vi "EnableCell.vi"(0 "SingleValMenuCol in":refnum<class "SingleValMenuCol.lvclass">, 5 "Cell Position":T1, 7 "Table Data in":string[][](array[string]), 9 "Table CtlRef In":refnum<vi>, 11 "error in (no error)":errorcluster) -> (4 "SingleValMenuCol out":refnum<class "SingleValMenuCol.lvclass">, 8 "Table Data out":string[][](array[string]), 10 "Table CtlRef Out":refnum<vi>, 15 "error out":errorcluster)   [LabVIEW 2013, in "SingleValMenuCol.lvclass"]
uses:
  SingleValMenuCol.lvclass
  <vilib>/Utility/miscctls.llb/LVRowAndColumnTypeDef.ctl
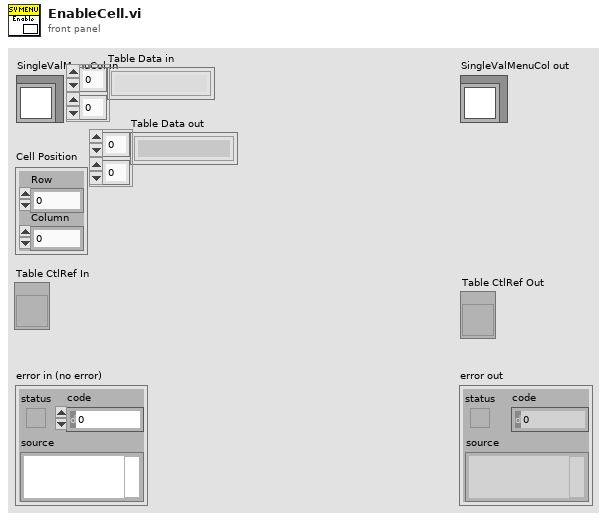
[diagram p1: front panel]
types:
  T1 = typedef "LVRowAndColumnTypeDef.ctl" = cluster{"Row":i32, "Column":i32}
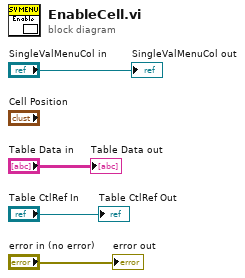
[diagram p0: block diagram]
diagram:
  "error out" <- "error in (no error)"
  "SingleValMenuCol out" <- "SingleValMenuCol in"
  "Table CtlRef Out" <- "Table CtlRef In"
  "Table Data out" <- "Table Data in"
